vi "TEST_IN.vi"(0 "NI_report输入":refnum<class "NI_report.lvclass">, 1 "试验员":string, 2 "编号":string, 3 "版本":string, 4 "检查员":string, 5 "错误输入（无错误）":errorcluster caption="error out", 7 "页码":string, 12 "_sheet_name":string, 13 "试验日期":string) -> (14 "NI_report输出":refnum<class "NI_report.lvclass">, 15 "试验员out":string, 18 "检查员out":string, 19 "错误输出":errorcluster caption="error out")   [LabVIEW 2013]
doc: "填写报表中的抬头，实验员，检验员，日期，页码等信息"
uses:
  <vilib>/Utility/NIReport.llb/NI_report.lvclass
  <vilib>/Utility/NIReport.llb/HTML Report Image Alignment.ctl
  <vilib>/Utility/NIReport.llb/Append Image to Report (path wrap).vi
  <vilib>/Utility/NIReport.llb/Append Report Text (str wrap).vi
  <vilib>/Utility/NIReport.llb/NI_ReportGenerationCore.lvlib
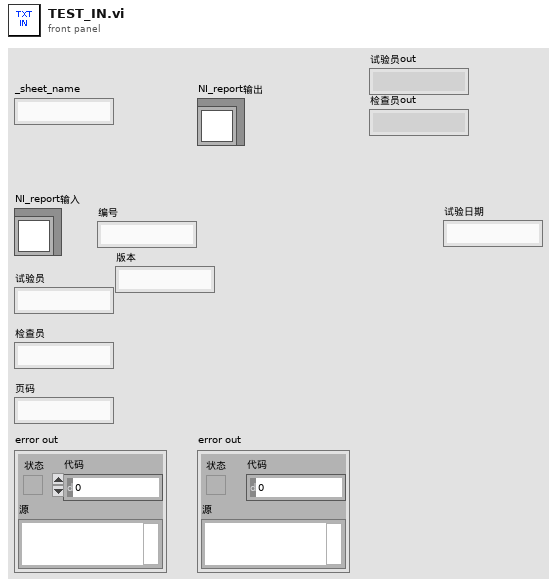
[diagram p1: front panel]
types:
  T1 = typedef "NI_ReportGenerationCore.lvlib/HTML Report Image Alignment.ctl" = enum16{"(default)", "LEFT", "RIGHT", "TOP", "TEXTTOP", "MIDDLE", "ABSMIDDLE", "BASELINE", "BOTTOM", "ABSBOTTOM"}
  T2 = cluster{"Italic":enum16{"Italic Unchanged", "Italic On", "Italic Off"}, "Strike Through":enum16{"Strike Through Unchanged", "Strike Through On", "Strike Through Off"}, "Underline":enum16{"Underline Unchanged", "Underline On", "Underline Off"}, "Bold":enum16{"Bold Unchanged", "Bold On", "Bold Off"}}
  T3 = cluster{"Charset (-1)":i16, "Weight (-1)":i16, "Name":string, "Size":string}
  T4 = cluster{"position (excel)":cluster{"row":i32, "column":i32}, string, "bookmark (word)":string}
  T5 = cluster{"position (Excel)":cluster{"row":i32, "column":i32}, string, "bookmark (word)":string}
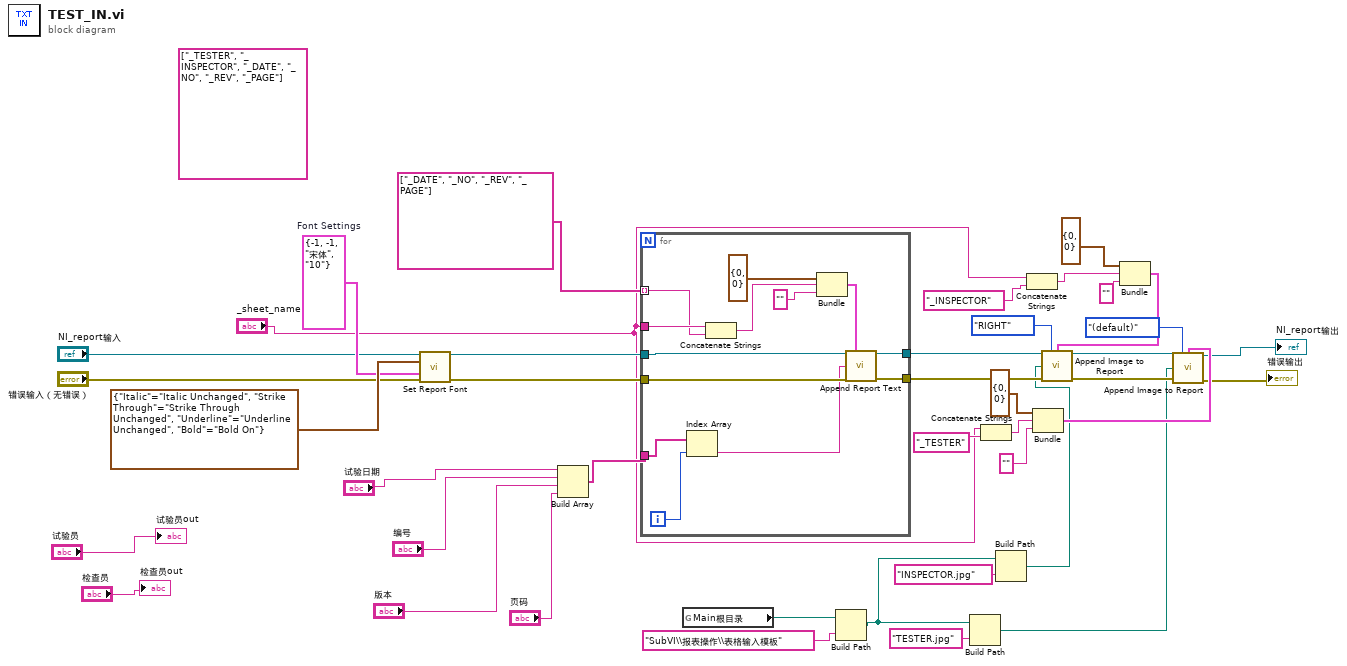
[diagram p0: block diagram]
diagram:
  (unwired) string[] ["_TESTER", "_INSPECTOR", "_DATE", "_NO", "_REV", "_PAGE"]
  w36 = T3 {"Charset (-1)"=-1, "Weight (-1)"=-1, "Name"="宋体", "Size"="10"}  # Font Settings
  n1 = call-dynamic "Set Report Font.vi"("report in"="NI_report输入", "text options"=T2 {"Italic"=enum."Italic Unchanged", "Strike Through"=enum."Strike Through Unchanged", "Underline"=enum."Underline Unchanged", "Bold"=enum."Bold On"}, "font settings"=w36, "error in (no error)"="错误输入（无错误）") -> ("report out"=w33:refnum<class "NI_report.lvclass">, "error out"=w32:errorcluster)  [unwired: 9 in, 1 out]
  n2 = Build Array("试验日期", "编号", "版本", "页码") -> (w40:string[])
  n3 = for {
    tunnel: string[] ["_DATE", "_NO", "_REV", "_PAGE"] -> [w52] mode=indexing
    tunnel: "_sheet_name" -> [w53]
    tunnel: w40 -> [w43]
    tunnel: w33 -> [w47]
    tunnel: w32 -> [w46]
    tunnel: [w45] -> w27
    tunnel: [w44] -> w26
    i -> [w42]
    n4 = Index Array(array=w43, index=w42) -> (element=w41:string)
    n5 = Concatenate Strings(w53, w52) -> (w49:string)
    n6 = Bundle("position (excel)"=cluster{"row":i32, "column":i32} {"row"=0, "column"=0}, w49, "bookmark (word)"="") -> (w48:T4)  [unwired: 1 in]
    n7 = call-poly <vilib>:"Append Report Text.vi"("report in"=w47, "MS Office parameters"=w48, "text"=w41, "error in (no error)"=w46) -> ("report out"=w45:refnum<class "NI_report.lvclass">, "error out"=w44:errorcluster)  [unwired: 8 in, 2 out]
  }
  n8 = global read "Main根目录.vi" "Main根目录"() -> (w1:path)
  n9 = Build Path(base path=w1, name or relative path="SubVI\\报表操作\\表格输入模板" ("名称或相对路径")) -> (appended path=w2:path)
  n10 = Build Path(base path=w2, name or relative path="TESTER.jpg" ("名称或相对路径")) -> (appended path=w10:path)
  n11 = Concatenate Strings("_sheet_name", "_TESTER" ("bookmark (word)")) -> (w21:string)
  n12 = Build Path(base path=w2, name or relative path="INSPECTOR.jpg" ("名称或相对路径")) -> (appended path=w8:path)
  n13 = Concatenate Strings("_sheet_name", "_INSPECTOR" ("bookmark (word)")) -> (w18:string)
  n14 = Bundle("position (Excel)"=cluster{"row":i32, "column":i32} {"row"=0, "column"=0}, w21, "bookmark (word)"="") -> (w20:T5)  [unwired: 1 in]
  n15 = Bundle("position (Excel)"=cluster{"row":i32, "column":i32} {"row"=0, "column"=0}, w18, "bookmark (word)"="") -> (w7:T5)  [unwired: 1 in]
  n16 = call-poly <vilib>:"Append Image to Report.vi"("report in"=w27, "alignment (default)"=HTML_Report_Image_Alignment."RIGHT", "MS Office parameters"=w7, "path or URL of image"=w8, "error in (no error)"=w26) -> ("report out"=w16:refnum<class "NI_report.lvclass">, "error out"=w15:errorcluster)  [unwired: 7 in, 2 out]
  n17 = call-poly <vilib>:"Append Image to Report.vi"("report in"=w16, "alignment (default)"=HTML_Report_Image_Alignment."(default)", "MS Office parameters"=w20, "path or URL of image"=w10, "error in (no error)"=w15) -> ("report out"=→"NI_report输出":refnum<class "NI_report.lvclass">, "error out"=→"错误输出":errorcluster)  [unwired: 7 in, 2 out]
  "试验员out" <- "试验员"
  "检查员out" <- "检查员"
